vi "Constructor.vi"(7 "VISA resource name":refnum<visa-resource-name>, 8 "error in (no error)":errorcluster, 9 "Device Type":u8, 10 "Tag ID":u32, 11 "Brooks MFC in":refnum<class "Brooks MFC.lvclass">) -> (0 "error out":errorcluster, 3 "Brooks MFC out":refnum<class "Brooks MFC.lvclass">)   [LabVIEW 2016, in "Brooks MFC.lvclass"]
uses:
  Brooks MFC.lvclass
  Brooks MFC.lvclass/Brooks MFC.ctl
  <vilib>/Instr/_visa.llb/VISA Configure Serial Port (Instr).vi
panel:
  # "Watch Out: \nIf \n     TAG ID == XXXXX00X\nThen\n     TAG ID in LABVIEW == XXXXX0X"
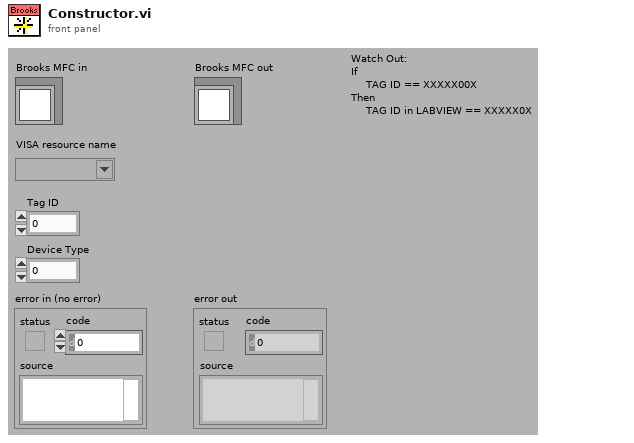
[diagram p1: front panel]
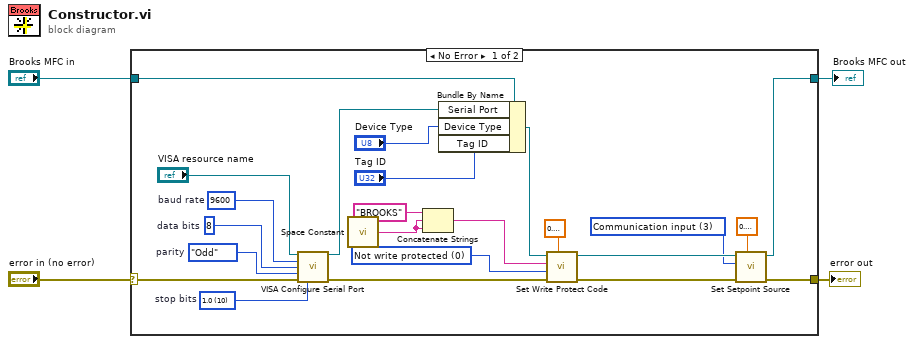
[diagram p0: block diagram]
diagram:
  n1 = case shown="No Error" "error in (no error)" {
    selector: "error in (no error)" -> [w23 w29]
    tunnel: [w5 w29] -> w3
    tunnel: [w6 w28] -> w1
    tunnel: "Brooks MFC in" -> [w22 w28]
    frame No Error {
      w7 = u8 3 items=["Undefined", "0..5 volt or 0..20mA input", "1..5 volt or 4..20mA input", "Communication input"] ("setpoint source")
      w16 = u8 0 items=["Not write protected", "Write protected", "Undefined"] ("Write Protect Code")
      w24 = u16 10 items=["1.0"=10, "1.5"=15, "2.0"=20]  # stop bits
      w25 = enum16{"None", "Odd", "Even", "Mark", "Space"}."Odd"  # parity
      w26 = u16 8  # data bits
      w27 = u32 9600  # baud rate
      n2 = call-poly "VISA Configure Serial Port"("VISA resource name"="VISA resource name", "baud rate (9600)"=w27, "data bits (8)"=w26, "parity (0:none)"=w25, "error in (no error)"=w23, "stop bits (10: 1 bit)"=w24) -> ("VISA resource name out"=w18:refnum<visa-resource-name>, "error out"=w11:errorcluster)  [unwired: 8 in]
      n3 = call <vilib>:"Space Constant.vi"() -> ("String"=w14:string)
      n4 = Concatenate Strings("BROOKS" ("string"), w14, w14) -> (w13:string)
      n5 = Bundle By Name(cluster=w22, "Serial Port"=w18, "Device Type"="Device Type", "Tag ID"="Tag ID") -> (w17:refnum<class "Brooks MFC.lvclass">)
      n6 = call "Set Write Protect Code.vi"("listen period"=sgl 0.1, "error in"=w11, "Write Protect Code"=w16, "Password"=w13, "Brooks MFC in"=w17) -> ("error out"=w10:errorcluster, "Brooks MFC out"=w9:refnum<class "Brooks MFC.lvclass">)  [unwired: 4 in, 1 out]
      n7 = call "Set Setpoint Source.vi"("listen period"=sgl 0.1, "error in"=w10, "setpoint source"=w7, "Brooks MFC in"=w9) -> ("error out"=w5:errorcluster, "Brooks MFC out"=w6:refnum<class "Brooks MFC.lvclass">)  [unwired: 5 in, 1 out]
    }
    frame Error {
    }
  }
  "error out" <- w3
  "Brooks MFC out" <- w1
